vi "Proceed.vi"(7 "component is ready (Y)":bool=TRUE, 8 "error in (no error)":errorcluster, 10 "ProceedMessage":refnum<class "ProceedMessage.lvclass">, 11 "Tomo in":refnum<class "Tomo.lvclass">) -> (0 "error out":errorcluster, 2 "all observers are ready?":bool, 3 "Tomo out":refnum<class "Tomo.lvclass">)   [LabVIEW 2012, in "Tomo.lvclass"]
uses:
  Tomo.lvclass
  <vilib>/Distrio/Murmex/ProceedMessage/ProceedMessage.lvclass
  <vilib>/Distrio/Murmex/StopMessage/StopMessage.lvclass
  Tomo.lvclass/Tomo.ctl
  <vilib>/Distrio/Murmex/GenericMessage/GenericMessage.lvclass
  Current activity.ctl
  <vilib>/Distrio/Murmex/StartMessage/StartMessage.lvclass
  <vilib>/Distrio/Murmex/StartMessage/run mode enum.ctl
  <vilib>/Distrio/Murmex/Murmex/Murmex.lvclass
  <vilib>/Distrio/Murmex/Message/Add or replace parameter.vi
  <vilib>/Distrio/Murmex/Message/Message.lvclass
panel:
  # "This method is called when the PROCEED\ntrigger is sent. \n\nOverride this method when your component needs to\nrespond to this trigger. \n\nCall parent for proper implementation"
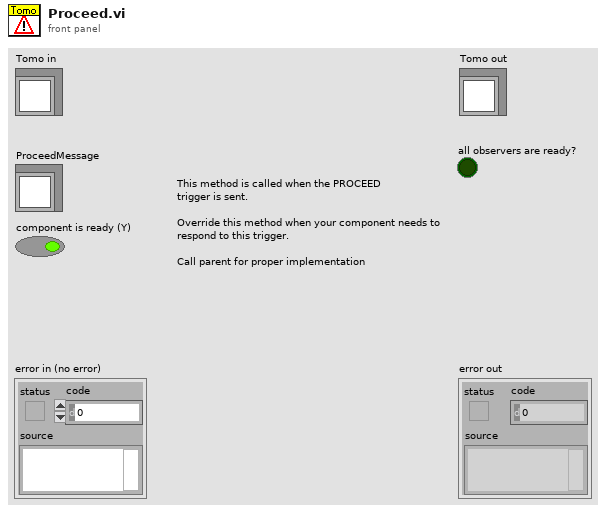
[diagram p1: front panel]
types:
  T1 = typedef "Tomo.lvclass/Current activity.ctl" = enum16{"Idle", "Inter-stack motion", "Pre-tomo calculation", "Stack acquisition", "Stack preparation", "Pre-tomo stack acq", "Pre-tomo inter-stack"}
  T2 = typedef "Murmex.lvlib/StartMessage.lvclass/run mode enum.ctl" = enum16{"infinite", "finite"}
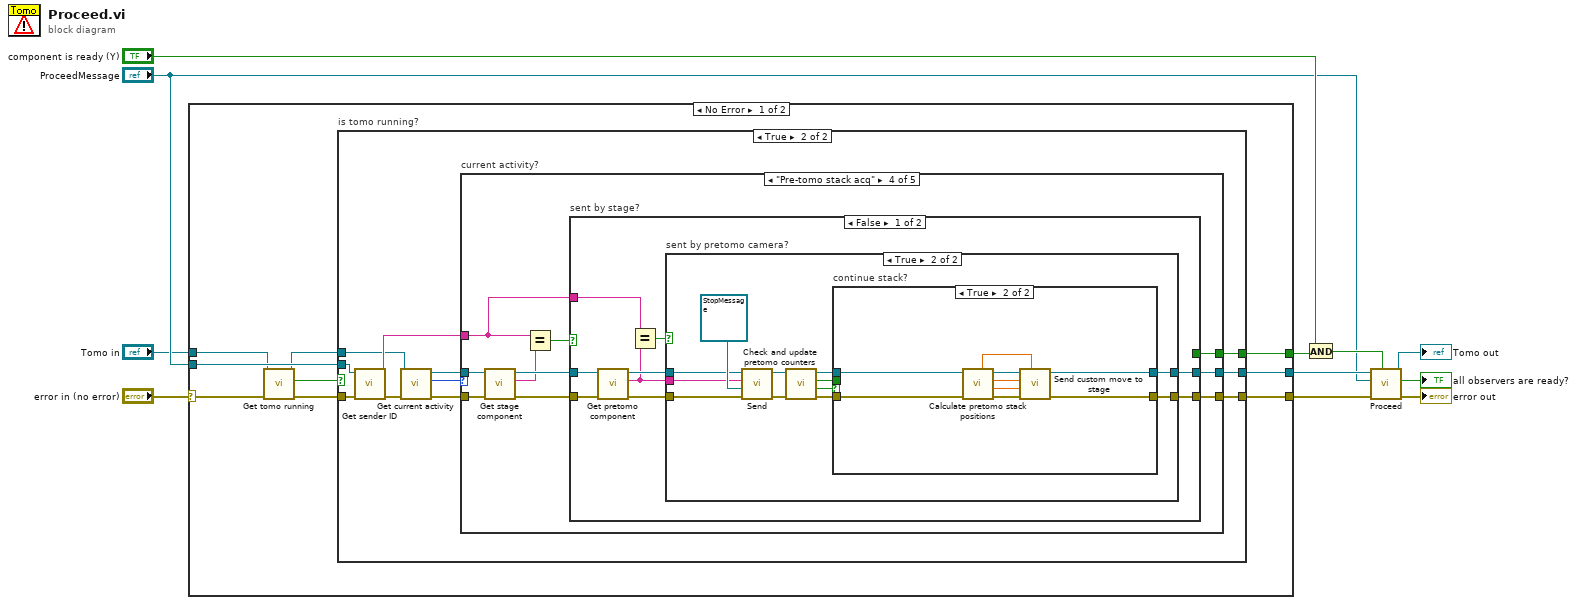
[diagram p0: block diagram]
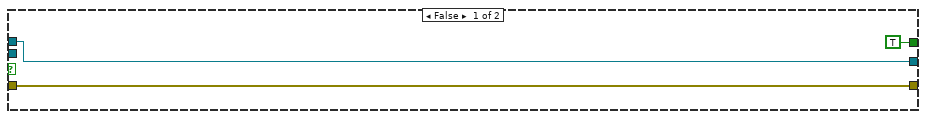
[diagram p2: hidden frame]
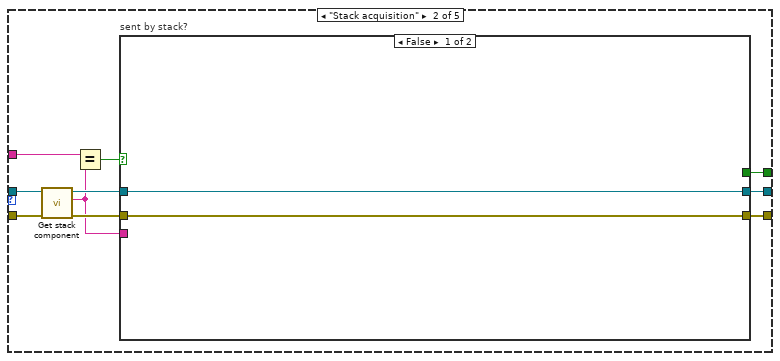
[diagram p4: hidden frame]
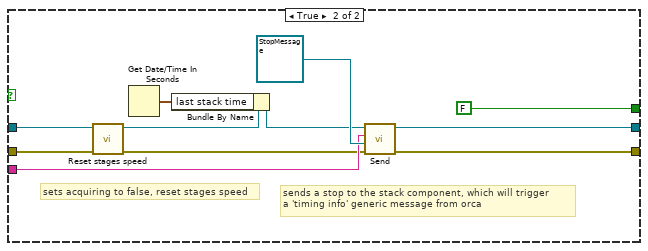
[diagram p5: hidden frame]
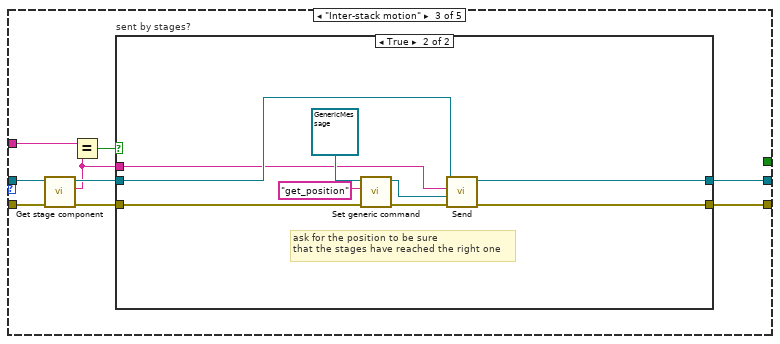
[diagram p6: hidden frame]
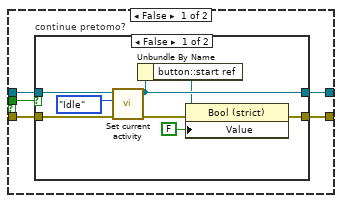
[diagram p9: hidden frame]
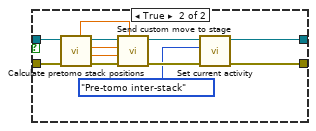
[diagram p10: hidden frame]
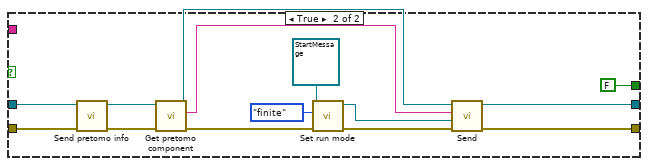
[diagram p11: hidden frame]
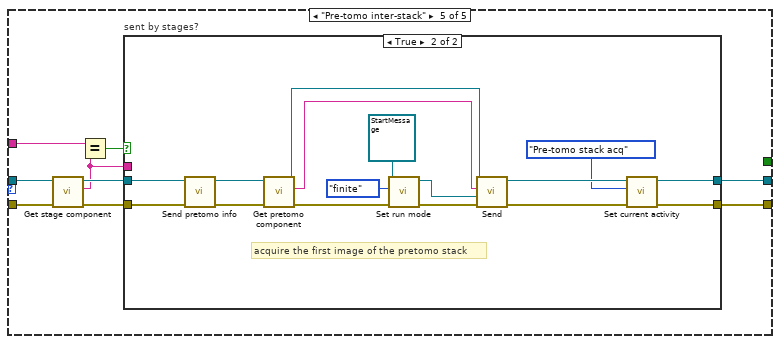
[diagram p12: hidden frame]
diagram:
  n1 = case shown="No Error" "error in (no error)" {
    selector: "error in (no error)" -> [w20 w189]
    tunnel: [w17 w189] -> w10
    tunnel: [w18 w188] -> w9
    tunnel: "ProceedMessage" -> [w19 _]
    tunnel: "Tomo in" -> [w14 w188]
    tunnel: [w16 _] -> w1
    frame No Error {
      n2 = call-dynamic "Get tomo running.vi"("error in (no error)"=w20, "Tomo in"=w14) -> ("error out"=w15:errorcluster, "tomo running?"=w12:bool, "Tomo out"=w13:refnum<class "Tomo.lvclass">)  [unwired: 7 in]
      n3 = case "is tomo running?" shown="True" w12 {
        tunnel: w15 -> [w22 w34]
        tunnel: w19 -> [_ w33]
        tunnel: w13 -> [w23 w27]
        tunnel: [w23 w31] -> w18
        tunnel: [w22 w30] -> w17
        tunnel: [TRUE w29] -> w16
        frame False {
        }
        frame True {
          n4 = call <vilib>:"Get sender ID.vi"("error in (no error)"=w34, "Message in"=w33) -> ("error out"=w28:errorcluster, "sender"=w32:string)  [unwired: 7 in, 1 out]
          n5 = call-dynamic "Get current activity.vi"("error in (no error)"=w28, "Tomo in"=w27) -> ("error out"=w25:errorcluster, "Current activity"=w24:T1, "Tomo out"=w26:refnum<class "Tomo.lvclass">)  [unwired: 7 in]
          n6 = case "current activity?" shown="\"Pre-tomo stack acq\"" w24 {
            tunnel: w32 -> [_ w41 w66 w80 w163]
            tunnel: w25 -> [w35 w43 w67 w85 w165]
            tunnel: w26 -> [w36 w42 w68 w83 w164]
            tunnel: [w36 w46 w62 w87 w162] -> w31
            tunnel: [w35 w45 w61 w86 w161] -> w30
            tunnel: [_ w44 _ w88 _] -> w29
            frame "Idle", Default {
            }
            frame "Stack acquisition" {
              n7 = call-dynamic "Get stack component.vi"("error in (no error)"=w43, "Tomo in"=w42) -> ("error out"=w38:errorcluster, "stack component"=w37:string, "Tomo out"=w39:refnum<class "Tomo.lvclass">)  [unwired: 7 in]
              n8 = Equal?(x=w41, y=w37) -> (x = y?=w40:bool)
              n9 = case "sent by stack?" shown="False" w40 {
                tunnel: w39 -> [w48 w52]
                tunnel: w38 -> [w47 w51]
                tunnel: [w48 w54] -> w46
                tunnel: [w47 w53] -> w45
                tunnel: w37 -> [_ w58]
                tunnel: [_ FALSE] -> w44
                frame False {
                }
                frame True {
                  # "sends a stop to the stack component, which will trigger\na 'timing info' generic message from orca"
                  # "sets acquiring to false, reset stages speed"
                  n10 = call-dynamic "Reset stages speed.vi"("error in (no error)"=w51, "Tomo in"=w52) -> ("error out"=w56:errorcluster, "Tomo out"=w57:refnum<class "Tomo.lvclass">)  [unwired: 8 in]
                  n11 = Get Date/Time In Seconds() -> (seconds since 1Jan1904=w49:timestamp)
                  n12 = Bundle By Name(cluster=w57, "last stack time"=w49) -> (w50:refnum<class "Tomo.lvclass">)
                  n13 = call <vilib>:"Send.vi"("error in (no error)"=w56, "Message"=refnum<class "StopMessage.lvclass"> refnum ("Message in"), "recipient"=w58, "Murmex in"=w50) -> ("error out"=w53:errorcluster, "Murmex out"=w54:refnum<class "Tomo.lvclass">)  [unwired: 6 in]
                }
              }
            }
            frame "Inter-stack motion" {
              n14 = call-dynamic "Get stage component.vi"("error in (no error)"=w67, "Tomo in"=w68) -> ("error out"=w64:errorcluster, "stage component"=w60:string, "Tomo out"=w63:refnum<class "Tomo.lvclass">)  [unwired: 7 in]
              n15 = Equal?(x=w66, y=w60) -> (x = y?=w65:bool)
              n16 = case "sent by stages?" shown="True" w65 {
                tunnel: w64 -> [w69 w75]
                tunnel: w63 -> [w70 w74]
                tunnel: [w70 w73] -> w62
                tunnel: [w69 w72] -> w61
                tunnel: w60 -> [_ w71]
                frame False {
                  # "does nothing. This might be a relayed proceed\nwhen the stages have moved to the starting position of \na stack"
                }
                frame True {
                  # "ask for the position to be sure\nthat the stages have reached the right one"
                  n17 = call <vilib>:"Set generic command.vi"("error in (no error)"=w75, "generic command"="get_position", "GenericMessage in"=refnum<class "GenericMessage.lvclass"> refnum ("Distrio Murmex 1.2:GenericMessage")) -> ("error out"=w77:errorcluster, "GenericMessage out"=w76:refnum<class "GenericMessage.lvclass">)  [unwired: 7 in]
                  n18 = call <vilib>:"Send.vi"("error in (no error)"=w77, "Message"=w76, "recipient"=w71, "Murmex in"=w74) -> ("error out"=w72:errorcluster, "Murmex out"=w73:refnum<class "Tomo.lvclass">)  [unwired: 6 in]
                }
              }
            }
            frame "Pre-tomo stack acq" {
              n19 = call-dynamic "Get stage component.vi"("error in (no error)"=w85, "Tomo in"=w83) -> ("error out"=w84:errorcluster, "stage component"=w81:string, "Tomo out"=w82:refnum<class "Tomo.lvclass">)  [unwired: 7 in]
              n20 = Equal?(x=w80, y=w81) -> (x = y?=w89:bool)
              n21 = case "sent by stage?" shown="False" w89 {
                tunnel: w82 -> [w97 w148]
                tunnel: w84 -> [w98 w150]
                tunnel: [w92 w152] -> w87
                tunnel: [w91 w151] -> w86
                tunnel: [_ FALSE] -> w88
                tunnel: w80 -> [w95 _]
                frame False {
                  n22 = call-dynamic "Get pretomo component.vi"("error in (no error)"=w98, "Tomo in"=w97) -> ("error out"=w93:errorcluster, "pretomo camera component"=w90:string, "Tomo out"=w94:refnum<class "Tomo.lvclass">)  [unwired: 7 in]
                  n23 = Equal?(x=w95, y=w90) -> (x = y?=w96:bool)
                  n24 = case "sent by pretomo camera?" shown="True" w96 {
                    tunnel: w94 -> [w100 w105]
                    tunnel: w93 -> [w99 w103]
                    tunnel: [w100 w109] -> w92
                    tunnel: [w99 w108] -> w91
                    tunnel: w90 -> [_ w101]
                    frame False {
                    }
                    frame True {
                      n25 = call <vilib>:"Send.vi"("error in (no error)"=w103, "Message"=refnum<class "StopMessage.lvclass"> refnum ("Message in"), "recipient"=w101, "Murmex in"=w105) -> ("error out"=w102:errorcluster, "Murmex out"=w104:refnum<class "Tomo.lvclass">)  [unwired: 6 in]
                      n26 = call-dynamic "Check and update pretomo counters.vi"("error in (no error)"=w102, "Tomo in"=w104) -> ("error out"=w111:errorcluster, "continue stack?"=w112:bool, "continue acquiring?"=w107:bool, "Tomo out"=w110:refnum<class "Tomo.lvclass">)  [unwired: 6 in]
                      n27 = case "continue stack?" shown="True" w112 {
                        tunnel: w111 -> [w115 w141]
                        tunnel: w110 -> [w116 w140]
                        tunnel: [w113 w139] -> w109
                        tunnel: [w114 w138] -> w108
                        tunnel: w107 -> [w117 _]
                        frame False {
                          n28 = case "continue pretomo?" shown="False" w117 {
                            tunnel: w116 -> [w124 w132]
                            tunnel: w115 -> [w123 w131]
                            tunnel: [w119 w129] -> w114
                            tunnel: [w122 w127] -> w113
                            frame False {
                              n29 = call-dynamic "Set current activity.vi"("error in (no error)"=w123, "Current activity"=Current_activity."Idle", "Tomo in"=w124) -> ("error out"=w120:errorcluster, "Tomo out"=w122:refnum<class "Tomo.lvclass">)  [unwired: 7 in]
                              n30 = Unbundle By Name(w122) -> ("button::start ref"=w121:refnum<vi>)
                              n31 = property class="Bool (strict)"(reference=w121, error in=w120, "Value"=FALSE) -> (error out=w119:errorcluster)  [unwired: 1 out]
                            }
                            frame True {
                              n32 = call-dynamic "Calculate pretomo stack positions.vi"("error in (no error)"=w131, "Tomo in"=w132) -> ("error out"=w136:errorcluster, "Y pos"=w133:dbl[unit], "X pos"=w134:dbl[unit], "Tomo out"=w137:refnum<class "Tomo.lvclass">, "Z pos"=w135:dbl[unit])  [unwired: 5 in]
                              n33 = call-dynamic "Send custom move to stage.vi"("Z pos"=w135, "error in (no error)"=w136, "Y pos"=w133, "X pos"=w134, "Tomo in"=w137) -> ("error out"=w130:errorcluster, "Tomo out"=w128:refnum<class "Tomo.lvclass">)  [unwired: 5 in]
                              n34 = call-dynamic "Set current activity.vi"("error in (no error)"=w130, "Current activity"=Current_activity."Pre-tomo inter-stack", "Tomo in"=w128) -> ("error out"=w129:errorcluster, "Tomo out"=w127:refnum<class "Tomo.lvclass">)  [unwired: 7 in]
                            }
                          }
                        }
                        frame True {
                          n35 = call-dynamic "Calculate pretomo stack positions.vi"("error in (no error)"=w141, "Tomo in"=w140) -> ("error out"=w145:errorcluster, "Y pos"=w142:dbl[unit], "X pos"=w143:dbl[unit], "Tomo out"=w146:refnum<class "Tomo.lvclass">, "Z pos"=w144:dbl[unit])  [unwired: 5 in]
                          n36 = call-dynamic "Send custom move to stage.vi"("Z pos"=w144, "error in (no error)"=w145, "Y pos"=w142, "X pos"=w143, "Tomo in"=w146) -> ("error out"=w138:errorcluster, "Tomo out"=w139:refnum<class "Tomo.lvclass">)  [unwired: 5 in]
                        }
                      }
                    }
                  }
                }
                frame True {
                  n37 = call-dynamic "Send pretomo info.vi"("error in (no error)"=w150, "Tomo in"=w148) -> ("error out"=w149:errorcluster, "Tomo out"=w147:refnum<class "Tomo.lvclass">)  [unwired: 8 in]
                  n38 = call-dynamic "Get pretomo component.vi"("error in (no error)"=w149, "Tomo in"=w147) -> ("error out"=w153:errorcluster, "pretomo camera component"=w155:string, "Tomo out"=w154:refnum<class "Tomo.lvclass">)  [unwired: 7 in]
                  n39 = call <vilib>:"Set run mode.vi"("error in (no error)"=w153, "run mode"=run_mode_enum."finite", "StartMessage in"=refnum<class "StartMessage.lvclass"> refnum ("Message in")) -> ("error out"=w157:errorcluster, "StartMessage out"=w156:refnum<class "StartMessage.lvclass">)  [unwired: 7 in]
                  n40 = call <vilib>:"Send.vi"("error in (no error)"=w157, "Message"=w156, "recipient"=w155, "Murmex in"=w154) -> ("error out"=w151:errorcluster, "Murmex out"=w152:refnum<class "Tomo.lvclass">)  [unwired: 6 in]
                }
              }
            }
            frame "Pre-tomo inter-stack" {
              n41 = call-dynamic "Get stage component.vi"("error in (no error)"=w165, "Tomo in"=w164) -> ("error out"=w168:errorcluster, "stage component"=w166:string, "Tomo out"=w167:refnum<class "Tomo.lvclass">)  [unwired: 7 in]
              n42 = Equal?(x=w163, y=w166) -> (x = y?=w169:bool)
              n43 = case "sent by stages?" shown="True" w169 {
                tunnel: w168 -> [w170 w175]
                tunnel: w167 -> [w171 w173]
                tunnel: [w171 w184] -> w162
                tunnel: [w170 w186] -> w161
                tunnel: w166 -> [_ _]
                frame False {
                  # "does nothing. This might be a relayed proceed\nwhen the stages have moved to the starting position of \na stack"
                }
                frame True {
                  # "acquire the first image of the pretomo stack"
                  n44 = call-dynamic "Send pretomo info.vi"("error in (no error)"=w175, "Tomo in"=w173) -> ("error out"=w174:errorcluster, "Tomo out"=w172:refnum<class "Tomo.lvclass">)  [unwired: 8 in]
                  n45 = call-dynamic "Get pretomo component.vi"("error in (no error)"=w174, "Tomo in"=w172) -> ("error out"=w176:errorcluster, "pretomo camera component"=w178:string, "Tomo out"=w177:refnum<class "Tomo.lvclass">)  [unwired: 7 in]
                  n46 = call <vilib>:"Set run mode.vi"("error in (no error)"=w176, "run mode"=run_mode_enum."finite", "StartMessage in"=refnum<class "StartMessage.lvclass"> refnum ("Message in")) -> ("error out"=w180:errorcluster, "StartMessage out"=w179:refnum<class "StartMessage.lvclass">)  [unwired: 7 in]
                  n47 = call <vilib>:"Send.vi"("error in (no error)"=w180, "Message"=w179, "recipient"=w178, "Murmex in"=w177) -> ("error out"=w187:errorcluster, "Murmex out"=w185:refnum<class "Tomo.lvclass">)  [unwired: 6 in]
                  n48 = call-dynamic "Set current activity.vi"("error in (no error)"=w187, "Current activity"=Current_activity."Pre-tomo stack acq", "Tomo in"=w185) -> ("error out"=w186:errorcluster, "Tomo out"=w184:refnum<class "Tomo.lvclass">)  [unwired: 7 in]
                }
              }
            }
          }
        }
      }
    }
    frame Error {
    }
  }
  n49 = And(x="component is ready (Y)", y=w1) -> (x .and. y?=w5:bool)
  n50 = call-parent "Proceed.vi"("component is ready (Y)"=w5, "error in (no error)"=w10, "ProceedMessage"="ProceedMessage", "Murmex in"=w9) -> ("error out"=→"error out":errorcluster, "all observers are ready?"=→"all observers are ready?":bool, "Murmex out"=→"Tomo out":refnum<class "Tomo.lvclass">)  [unwired: 5 in]
